vi "Enum To String Array.vi"(11 "Interface Type":T1=enum."Serial Master") -> (3 "Strings":string[](array[string]))   [LabVIEW 2015]
uses:
  Shared/Controls/Interface Type.ctl
  Shared/Modbus Master Shared.lvlib
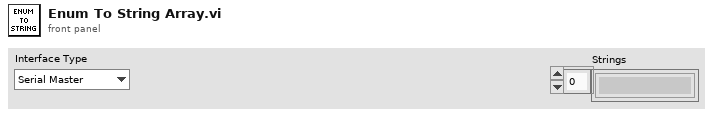
[diagram p1: front panel]
types:
  T1 = typedef "Modbus Master Shared.lvlib/Interface Type.ctl" = enum16{"TCP Master", "Serial Master"}
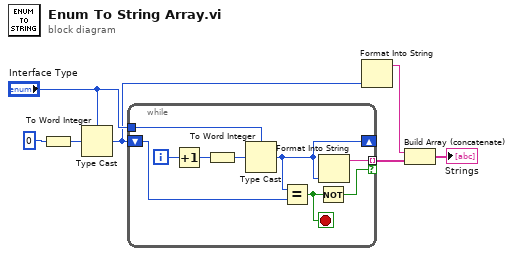
[diagram p0: block diagram]
diagram:
  n1 = To Word Integer(number=i16 0) -> (16bit integer=w7:i16)
  n2 = Type Cast(type="Interface Type", x=w7) -> (*(type *) &x=w4:T1)
  n3 = while {
    tunnel: "Interface Type" -> [w16]
    tunnel: [w14] -> w2 mode=indexing if=w8
    shift-right: [w11] -> _
    shift-left: w4 -> [w10]
    i -> [w12]
    stop <- w9 stop-if-true
    n4 = Increment(x=w12) -> (x+1=w13:i32)
    n5 = To Word Integer(number=w13) -> (16bit integer=w15:i16)
    n6 = Type Cast(type=w16, x=w15) -> (*(type *) &x=w11:T1)
    n7 = Equal?(x=w11, y=w10) -> (x = y?=w9:bool)
    n8 = Not(x=w9) -> (.not. x?=w8:bool)
    n9 = Format Into String(w11) -> (resulting string=w14:string)  [unwired: 3 in, 1 out]
  }
  n10 = Format Into String(w4) -> (resulting string=w3:string)  [unwired: 3 in, 1 out]
  n11 = Build Array (concatenate)(w3, w2) -> (→"Strings":string[])
